vi "counter 2.vi"() -> ()   [LabVIEW 2009]
panel:
  out "Compte total":i32
  out "Compte 2":i32
  out "total cumulatif":i32
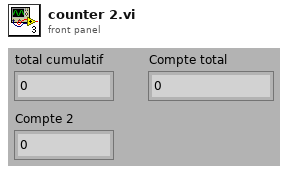
[diagram p1: front panel]
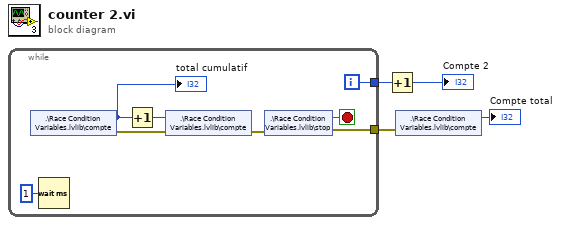
[diagram p0: block diagram]
diagram:
  n1 = while "Boucle While" {
    tunnel: [w10] -> w4
    tunnel: [w9] -> w1
    i -> [w10]
    stop <- w5 stop-if-true
    n2 = shared-variable ".\\Race Condition Variables.lvlib\\compte"() -> (w6:i32, error out=w12:errorcluster)  [unwired: 1 in]
    "total cumulatif" <- w6
    n3 = Wait (ms) ("Attendre (ms)")(milliseconds to wait=u32 1) -> ()  [unwired: 1 out]
    n4 = Increment ("Incrémenter")(x=w6) -> (x+1=w7:i32)
    n5 = shared-variable ".\\Race Condition Variables.lvlib\\compte"(w7, error in=w12) -> (error out=w11:errorcluster)
    n6 = shared-variable ".\\Race Condition Variables.lvlib\\stop"(error in=w11) -> (w5:bool, error out=w9:errorcluster)
  }
  n7 = Increment ("Incrémenter")(x=w4) -> (x+1=→"Compte 2":i32)
  n8 = shared-variable ".\\Race Condition Variables.lvlib\\compte"(error in=w1) -> (→"Compte total":i32)  [unwired: 1 out]
